vi "Clear All Configurations.vi"(8 "error in (no error)":errorcluster, 11 "Station Config in":refnum<class "Station Config.lvclass">) -> (0 "error out":errorcluster, 3 "Station Config out":refnum<class "Station Config.lvclass">)   [LabVIEW 2015, in "Station Config.lvlib" / "Station Config.lvclass"]
uses:
  Station Config.lvclass
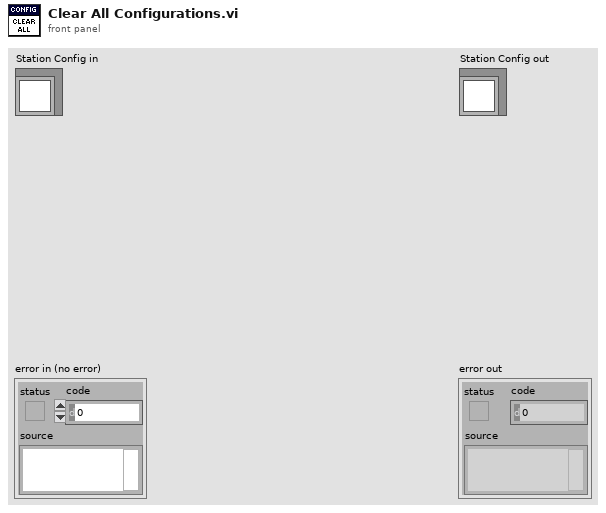
[diagram p1: front panel]
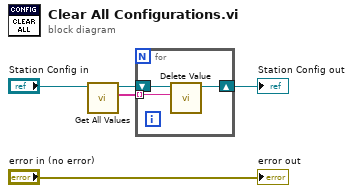
[diagram p0: block diagram]
diagram:
  n1 = call-dynamic "Get All Values.vi"("Registry in"="Station Config in") -> ("Keys"=w1:string[], "Registry out"=w3:refnum<class "Station Config.lvclass">)  [unwired: 7 in, 2 out]
  n2 = for {
    shift-right: [w7] -> w2
    shift-left: w3 -> [w8]
    tunnel: w1 -> [w6] mode=indexing
    n3 = call-dynamic "Delete Value.vi"("Key"=w6, "Registry in"=w8) -> ("Registry out"=w7:refnum<class "Station Config.lvclass">)  [unwired: 7 in, 2 out]
  }
  "Station Config out" <- w2
  "error out" <- "error in (no error)"
